vi "Close.vi"(8 "error in (no error)":errorcluster, 11 "MultiResponder in":refnum<class "MultiResponder.lvclass">) -> (0 "error out":errorcluster, 3 "MultiResponder out":refnum<class "MultiResponder.lvclass">)   [LabVIEW 2013, in "MultiResponder.lvclass"]
doc: "Closes all open references and reserved resources for the responder"
uses:
  MultiResponder.lvclass
  BaseResponder/BaseResponder.lvclass
  MultiResponder.lvclass/MultiResponder.ctl
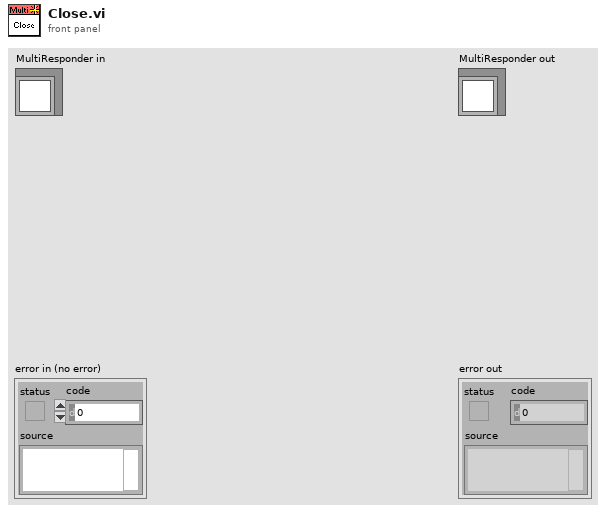
[diagram p1: front panel]
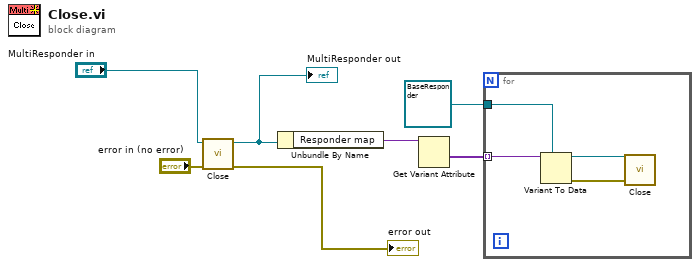
[diagram p0: block diagram]
diagram:
  n1 = call-parent "Close.vi"("error in (no error)"="error in (no error)", "BaseResponder in"="MultiResponder in") -> ("error out"=→"error out":errorcluster, "BaseResponder out"=w4:refnum<class "MultiResponder.lvclass">)  [unwired: 8 in]
  "MultiResponder out" <- w4
  n2 = Unbundle By Name(w4) -> ("Responder map"=w1:variant)
  n3 = Get Variant Attribute(Variant=w1) -> (values=w3:variant[])  [unwired: 3 in, 3 out]
  n4 = for {
    tunnel: w3 -> [w11] mode=indexing
    tunnel: refnum<class "BaseResponder.lvclass"> refnum ("BaseResponder.lvclass") -> [w10]
    n5 = Variant To Data(type=w10, Variant=w11) -> (data=w9:refnum<class "BaseResponder.lvclass">, error out=w8:errorcluster)  [unwired: 1 in]
    n6 = call-dynamic "Close.vi"("error in (no error)"=w8, "BaseResponder in"=w9) -> ()  [unwired: 8 in, 2 out]
  }
